vi "close channel.vi"(8 "error in":errorcluster, 11 "DAQ Config":T1) -> (0 "error out":errorcluster)   [LabVIEW 2017, in "Acquisition.lvlib"]
uses:
  Acquisition/Acquisition.lvlib
  Control/Config chanel.ctl
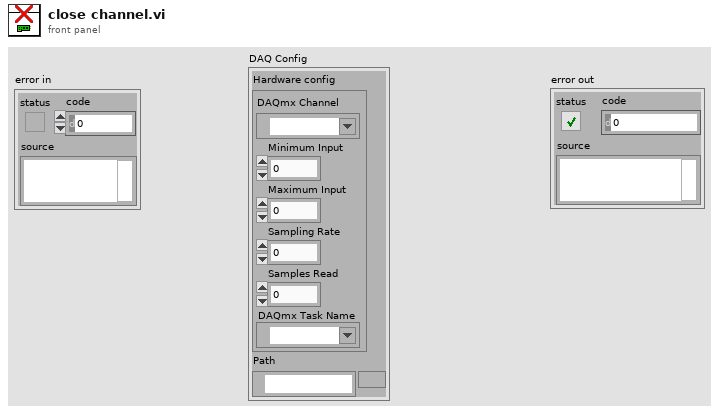
[diagram p1: front panel]
types:
  T1 = typedef "Config chanel.ctl" = cluster{"Hardware config":cluster{"DAQmx Channel":tag, "Minimum Input":dbl, "Maximum Input":dbl, "Sampling Rate":dbl, "Samples Read":dbl, "DAQmx Task Name":refnum<k21>}, "Path":path}
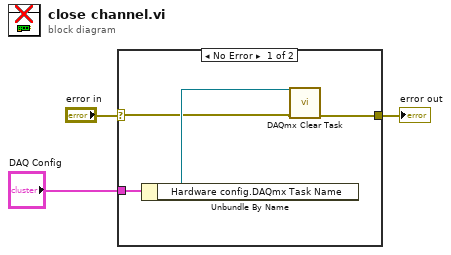
[diagram p0: block diagram]
diagram:
  n1 = case shown="No Error" "error in" {
    selector: "error in" -> [w4 w8]
    tunnel: [w7 w8] -> w2
    tunnel: "DAQ Config" -> [w6 _]
    frame No Error {
      n2 = Unbundle By Name(w6) -> ("Hardware config.DAQmx Task Name"=w5:refnum<k21>)
      n3 = call <vilib>:"DAQmx Clear Task.vi"("task in"=w5, "error in"=w4) -> ("error out"=w7:errorcluster)  [unwired: 13 in]
    }
    frame Error {
    }
  }
  "error out" <- w2
